vi "边界判断.vi"(5 "列":i32, 7 "行":i32, 8 "列索引":i32, 9 "行索引":i32, 10 "滤波器大小":i32) -> (2 "输出列索引":i32, 3 "输出行索引":i32)   [LabVIEW 2016]
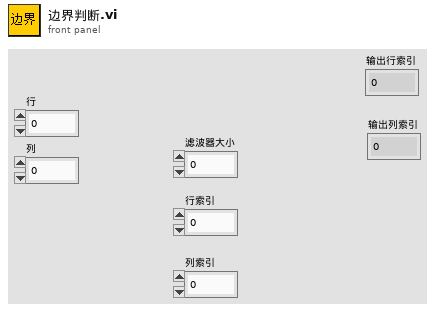
[diagram p1: front panel]
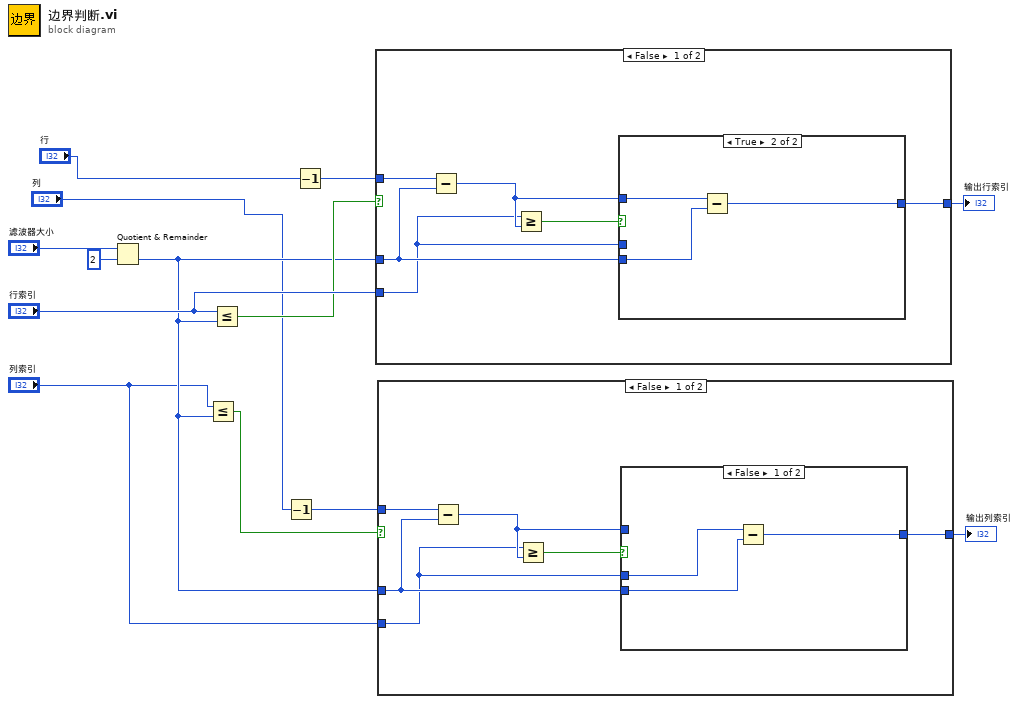
[diagram p0: block diagram]
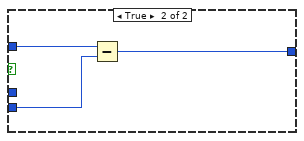
[diagram p2: hidden frame]
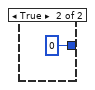
[diagram p3: hidden frame]
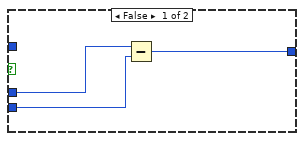
[diagram p4: hidden frame]
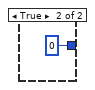
[diagram p5: hidden frame]
diagram:
  n1 = Quotient & Remainder(x="滤波器大小", y=2) -> (floor(x/y)=w6:i32)  [unwired: 1 out]
  n2 = Less Or Equal?(x="列索引", y=w6) -> (x <= y?=w7:bool)
  n3 = Less Or Equal?(x="行索引", y=w6) -> (x <= y?=w9:bool)
  n4 = Decrement(x="列") -> (x-1=w8:i32)
  n5 = Decrement(x="行") -> (x-1=w10:i32)
  n6 = case shown="False" w9 {
    tunnel: w10 -> [w19 _]
    tunnel: "行索引" -> [w14 _]
    tunnel: w6 -> [w16 _]
    tunnel: [w15 0] -> w4
    frame False {
      n7 = Subtract(x=w19, y=w16) -> (x-y=w17:i32)
      n8 = Greater Or Equal?(x=w14, y=w17) -> (x >= y?=w18:bool)
      n9 = case shown="True" w18 {
        tunnel: w17 -> [_ w25]
        tunnel: w16 -> [w21 w24]
        tunnel: [w20 w23] -> w15
        tunnel: w14 -> [w22 _]
        frame False {
          n10 = Subtract(x=w22, y=w21) -> (x-y=w20:i32)
        }
        frame True {
          n11 = Subtract(x=w25, y=w24) -> (x-y=w23:i32)
        }
      }
    }
    frame True {
    }
  }
  "输出行索引" <- w4
  n12 = case shown="False" w7 {
    tunnel: w8 -> [w32 _]
    tunnel: "列索引" -> [w27 _]
    tunnel: w6 -> [w29 _]
    tunnel: [w28 0] -> w3
    frame False {
      n13 = Subtract(x=w32, y=w29) -> (x-y=w30:i32)
      n14 = Greater Or Equal?(x=w27, y=w30) -> (x >= y?=w31:bool)
      n15 = case shown="False" w31 {
        tunnel: w30 -> [_ w38]
        tunnel: w29 -> [w34 w37]
        tunnel: [w33 w36] -> w28
        tunnel: w27 -> [w35 _]
        frame False {
          n16 = Subtract(x=w35, y=w34) -> (x-y=w33:i32)
        }
        frame True {
          n17 = Subtract(x=w38, y=w37) -> (x-y=w36:i32)
        }
      }
    }
    frame True {
    }
  }
  "输出列索引" <- w3
